vi "Kyriakakis_LabView_Software.vi"() -> ()   [LabVIEW 2012]
uses:
  <vilib>/MakerHub/LINX/LMH-LINX.lvlib
  <vilib>/MakerHub/LINX/Public/Peripherals/Digital/Digital Write N Chans.vi
panel:
  in  "Run Time           8":dbl min=0.0 step=60.0 format="%<%H:%M>t"
  in  "Run Time           7":dbl min=0.0 step=60.0 format="%<%H:%M>t"
  in  "Run Time           6":dbl min=0.0 step=60.0 format="%<%H:%M>t"
  in  "Run Time           5":dbl min=0.0 step=60.0 format="%<%H:%M>t"
  in  "Run Time           4":dbl min=0.0 step=60.0 format="%<%H:%M>t"
  in  "Run Time           3":dbl min=0.0 step=60.0 format="%<%H:%M>t"
  in  "Run Time           2":dbl min=0.0 step=60.0 format="%<%H:%M>t"
  in  "Run Time           1":dbl min=0.0 step=60.0 format="%<%H:%M>t"
  in  "Name/Notes":string
  in  "Pin #     8":u8=10 max=13 step=1
  out "Indicator         8":bool
  out "Cycle Time 8":dbl format="%<%H:%M>t"
  out "Frequency  8":dbl format="%#_3g mHz"
  in  "On/Off      8":bool
  out "On/Off indicator    8":bool
  in  "Time Off     8":dbl min=0.0 format="%#_4g min"
  in  "Time On    8":dbl min=0.0 format="%#_4g min"
  in  "Name/Notes":string
  in  "Pin #     7":u8=9 max=13 step=1
  out "Indicator         7":bool
  out "Cycle Time 7":dbl format="%<%H:%M>t"
  out "Frequency  7":dbl format="%#_3g mHz"
  in  "On/Off      7":bool
  out "On/Off indicator    7":bool
  in  "Time Off     7":dbl min=0.0 format="%#_2g min"
  in  "Time On    7":dbl min=0.0 format="%#_2g min"
  in  "Name/Notes":string
  in  "Pin #     6":u8=8 max=13 step=1
  out "Indicator         6":bool
  out "Cycle Time 6":dbl format="%<%H:%M>t"
  out "Frequency  6":dbl format="%#_3g mHz"
  in  "On/Off      6":bool
  out "On/Off indicator    6":bool
  in  "Time Off     6":dbl min=0.0 format="%#_2g min"
  in  "Time On    6":dbl min=0.0 format="%#_2g min"
  in  "Name/Notes":string
  in  "Pin #     5":u8=7 max=13 step=1
  out "Indicator         5":bool
  out "Cycle Time 5":dbl format="%<%H:%M>t"
  out "Frequency  5":dbl format="%#_3g mHz"
  in  "On/Off      5":bool
  out "On/Off indicator    5":bool
  in  "Time Off     5":dbl min=0.0 format="%#_2g min"
  in  "Time On    5":dbl min=0.0 format="%#_2g min"
  out "Connected":bool
  in  "?":bool
  in  "Name/Notes":string
  in  "Name/Notes":string
  in  "Name/Notes":string
  in  "Name/Notes":string
  in  "?":bool
  out "Run Complete":bool
  out "Time Has Elapsed":bool=TRUE
  out "Indicator         4":bool
  out "Cycle Time 4":dbl format="%<%H:%M>t"
  out "Frequency  4":dbl format="%#_3g mHz"
  in  "On/Off      4":bool
  out "On/Off indicator    4":bool
  in  "Time Off     4":dbl min=0.0 format="%#_2g min"
  in  "Time On    4":dbl min=0.0 format="%#_2g min"
  out "Indicator         3":bool
  out "Cycle Time 3":dbl format="%<%H:%M>t"
  out "Frequency  3":dbl format="%#_3g mHz"
  in  "On/Off      3":bool
  out "On/Off indicator    3":bool
  in  "Time Off     3":dbl min=0.0 format="%#_2g min"
  in  "Time On    3":dbl min=0.0 format="%#_2g min"
  in  "Pin #     4":u8=6 max=13 step=1
  in  "Pin #     3":i8=5 min=0 max=13 step=1
  in  "Pin #     2":u8=4 max=13 step=1
  out "Indicator         2":bool
  out "Cycle Time 2":dbl format="%<%H:%M>t"
  out "Frequency  2":dbl format="%#_3g mHz"
  in  "On/Off      2":bool
  out "On/Off indicator    2":bool
  in  "Time Off     2":dbl min=0.0 format="%#_2g min"
  in  "Time On    2":dbl min=0.0 format="%#_2g min"
  in  "Pin #     1":u8=3 max=13 step=1
  in  "Serial Port":refnum<visa-resource-name>
  out "Loop Rate (Hz)":u32
  out "Run Time":dbl format="%<%H:%M:%S>t"
  in  "Total Run Time \nH : M":dbl format="%<%M:%S>t"
  out "ACTIVE":bool
  in  "Start":bool
  out "Time till Start":dbl format="%<%H:%M:%S>t"
  in  "Start Delay\nH : M":dbl format="%<%M:%S>t"
  out "Total Elapsed Time":dbl format="%<%H:%M:%S>t"
  out "Indicator         1":bool
  out "Cycle Time 1":dbl format="%<%H:%M>t"
  out "Frequency  1":dbl format="%#_3g mHz"
  in  "On/Off      1":bool
  out "On/Off indicator    1":bool
  in  "Time Off     1":dbl min=0.0 format="%#_2g min"
  in  "Time On    1":dbl min=0.0 format="%#_2g min"
  # "Pin Controls:\nAll Time settings are given in Minutes\nKeep panel Off if not in use\nSelect pin you wish to use\nName/Notes can be edited for notes"
  # "Frequenices are in miliHertz (Cycles / 1000s)\nCycle Time is in Minutes\n% On is the Percentage of the On State\nIndicator indicaters if power is sent to light\nIf Individual Run times are 0, they default to total run time"
  # "Arduino Control Panel"
  # "Choose Serial Port from drop-down menu and click connect"
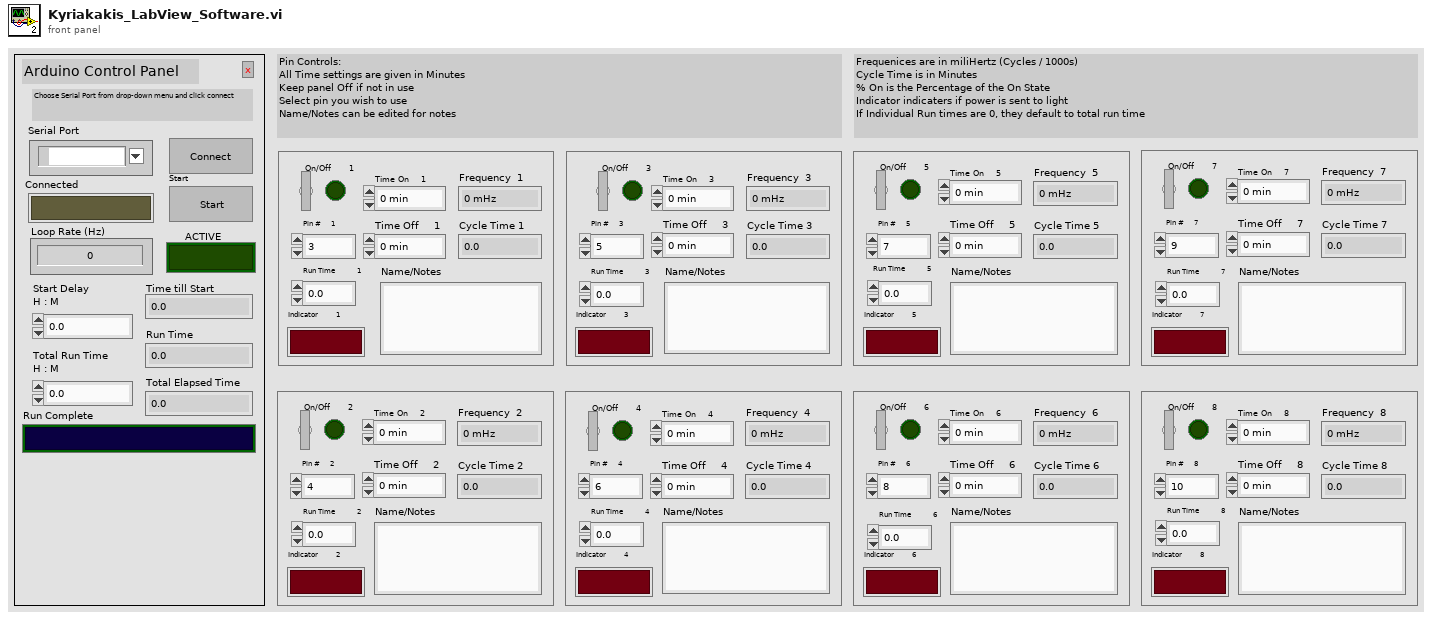
[diagram p1: front panel]
types:
  T1 = typedef "LMH-LINX.lvlib/LINX Ref.ctl" = cluster{"IO":T2, "Interface":T3, "LINX Device Config":T4}
  T2 = typedef "LMH-LINX.lvlib/Platform.ctl" = enum16{"Remote", "Local"}
  T3 = typedef "LMH-LINX.lvlib/Interface.ctl" = enum16{"Serial", "TCP"}
  T4 = typedef "LMH-LINX.lvlib/Device.lvlib/LINX Device Config.ctl" = cluster{"Interface":T3, "COM Port":refnum<visa-resource-name>, "TCP Configuration":T5, "Device Family":u8, "Device ID":u8, "Device Name":string, "TCP Ref":refnum<k5>, "Channels":T6}
  T5 = typedef "LMH-LINX.lvlib/Device.lvlib/TCP Config.ctl" = cluster{"IP Address":string, "Port":u16}
  T6 = typedef "LMH-LINX.lvlib/Channels.ctl" = cluster{"DI":u8[], "DO":u8[], "AI":u8[], "AO":u8[], "PWM":u8[], "QE":u8[], "UART":u8[], "I2C 2":u8[], "SPI":u8[], "CAN":u8[], "Servo":u8[], "AI Ref (V)":dbl, "AI Resolution (Bits)":u8, "AO Ref (V)":dbl, "AO Resolution (Bits)":u8}
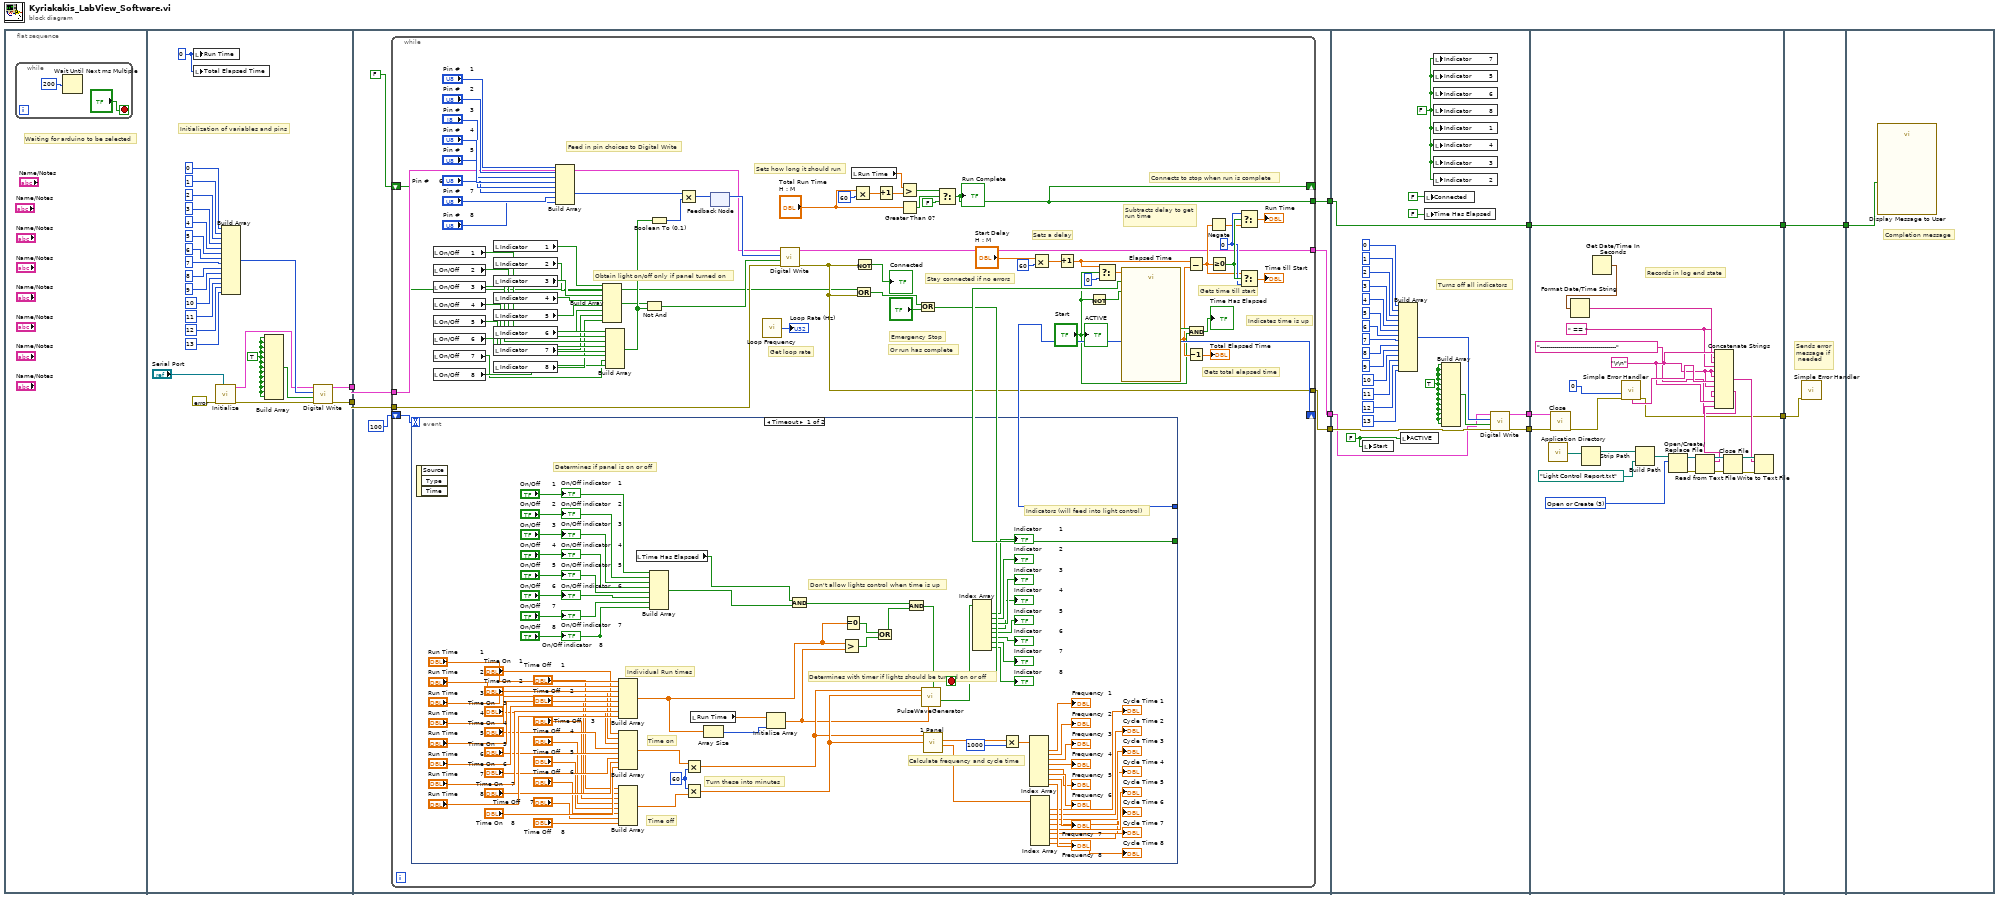
[diagram p0: block diagram]
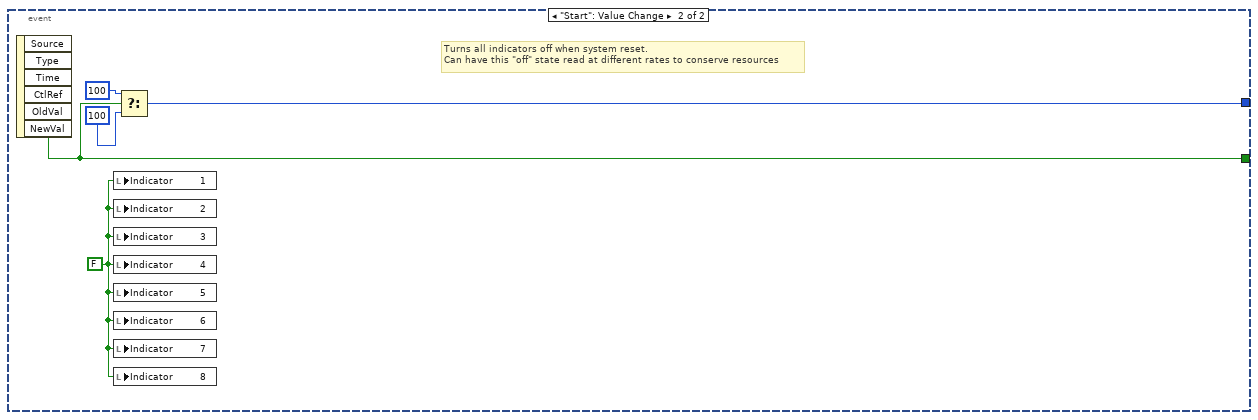
[diagram p2: hidden frame]
diagram:
  n1 = flat-sequence {
    tunnel: [w18] -> w7
    tunnel: [w17] -> w6
    tunnel: [w39] -> w11
    tunnel: [w40] -> w10
    tunnel: w7 -> [w44]
    tunnel: w6 -> [w43]
    tunnel: [w38] -> w5
    tunnel: w11 -> [w222]
    tunnel: w10 -> [w199]
    tunnel: [w220] -> w9
    tunnel: [w219] -> w8
    tunnel: w5 -> [w198]
    tunnel: [w198] -> w1
    tunnel: w9 -> [w248]
    tunnel: w8 -> [w247]
    tunnel: [w225] -> w4
    tunnel: [w224] -> w2
    tunnel: w1 -> [w224]
    tunnel: w4 -> [w250]
    tunnel: [w249] -> w3
    tunnel: w2 -> [w249]
    tunnel: w3 -> [w251]
    frame #0 {
      # "Waiting for arduino to be selected"
      n2 = while {
        stop <- "?" stop-if-true
        n3 = Wait Until Next ms Multiple(millisecond multiple=200) -> ()  [unwired: 1 out]
      }
    }
    frame #1 {
      w19 = TRUE
      w14 = 0
      # "Initialization of variables and pins"
      n4 = local write "Run Time"(w14) -> ()
      n5 = local write "Total Elapsed Time"(w14) -> ()
      n6 = call <vilib>:"Initialize.vi"("Serial Port"="Serial Port", "Error In"=errorcluster {"status"=FALSE, "code"=0, "source"=""}) -> ("Error Out"=w15:errorcluster, "LINX Resource"=w16:T1)  [unwired: 7 in, 1 out]
      n7 = Build Array(0, 1, 2, 3, 4, 5, 6, 7, 8, 9, 10, 11, 12, 13) -> (w20:i32[])
      n8 = Build Array(w19, w19, w19, w19, w19, w19, w19, w19, w19, w19, w19, w19, w19) -> (w35:bool[])
      n9 = call-poly <vilib>:"Digital Write.vi"("Error In"=w15, "Values"=w35, "DO Channels"=w20, "LINX Resource"=w16) -> ("Error Out"=w17:errorcluster, "LINX Resource"=w18:T1)  [unwired: 6 in]
    }
    frame #2 {
      n10 = while {
        shift-right: [w99] -> _
        shift-left: 100 -> [w98]
        tunnel: w43 -> [w87]
        tunnel: w44 -> [w49]
        tunnel: [w71] -> w39
        tunnel: [w86] -> w40
        shift-right: [w74] -> _
        shift-left: FALSE -> [w45]
        tunnel: [w74] -> w38
        stop <- w75 stop-if-true
        w108 = 0
        # "Or run has complete"
        # "Connects to stop when run is complete"
        # "Sets how long it should run"
        # "Gets time till start"
        # "Subtracts delay to get\nrun time"
        # "Sets a delay"
        # "Gets total elapsed time"
        # "Indicates time is up"
        # "Emergency Stop"
        # "Stay connected if no errors"
        # "Get loop rate"
        # "Obtain light on/off only if panel turned on"
        # "Feed in pin choices to Digital Write"
        n11 = event shown="[0] Timeout" {
          selector: _ -> [_ _]
          dyn-events: _ -> [_ _]
          timeout: w98 -> [_ _]
          tunnel: [_ w195] -> w99
          tunnel: [_ w194] -> w79
          event Timeout {
            w192 = 60
            # "Indicators (will feed into light control)"
            # "Determines with timer if lights should be turned on or off"
            # "Calculate frequency and cycle time"
            # "Turn these into minutes"
            # "Time off"
            # "Time on"
            # "Individual Run times"
            # "Don't allow lights control when time is up"
            # "Determines if panel is on or off"
            n12 = event-data() -> ()  [unwired: 1 in, 3 out]
            n13 = Build Array("Time On    1", "Time On    2", "Time On    3", "Time On    4", "Time On    5", "Time On    6", "Time On    7", "Time On    8") -> (w130:dbl[])
            n14 = Build Array("Run Time           1", "Run Time           2", "Run Time           3", "Run Time           4", "Run Time           5", "Run Time           6", "Run Time           7", "Run Time           8") -> (w118:dbl[])
            n15 = Build Array("Time Off     1", "Time Off     2", "Time Off     3", "Time Off     4", "Time Off     5", "Time Off     6", "Time Off     7", "Time Off     8") -> (w164:dbl[])
            n16 = local read "Time Has Elapsed"() -> (w121:bool)
            n17 = Build Array("On/Off      1", "On/Off      2", "On/Off      3", "On/Off      4", "On/Off      5", "On/Off      6", "On/Off      7", "On/Off      8") -> (w120:bool[])
            n18 = Multiply(x=w130, y=w192) -> (x*y=w145:dbl[])
            n19 = Multiply(x=w192, y=w164) -> (x*y=w146:dbl[])
            n20 = local read "Run Time"() -> (w142:dbl)
            n21 = Array Size(array=w118) -> (size(s)=w143:i32)
            n22 = Initialize Array(w142, w143) -> (w119:dbl[])
            n23 = And(x=w121, y=w120) -> (x .and. y?=w124:bool[])
            n24 = Greater?(x=w118, y=w119) -> (0:w190:bool[])
            n25 = Equal To 0?(x=w118) -> (x = 0?=w191:bool[])
            n26 = Or(x=w191, y=w190) -> (x .or. y?=w125:bool[])
            n27 = And(x=w124, y=w125) -> (x .and. y?=w144:bool[])
            n28 = call "PulseWaveGenerator.vi"("On/Off"=w144, "TIMER"=w119, "Time off (seconds)"=w146, "Time On (seconds)"=w145) -> ("Indicator"=w122:bool[])  [unwired: 6 in, 1 out]
            n29 = call "1 Panel.vi"("Time Off"=w146, "Time On"=w145) -> ("Cycle Time"=w155:dbl[], "Frequency"=w116:dbl[])  [unwired: 7 in, 1 out]
            n30 = Index Array(array=w122) -> (element #1=→"Indicator         1":bool, element #2=→"Indicator         2":bool, element #3=→"Indicator         3":bool, element #4=→"Indicator         4":bool, element #5=→"Indicator         5":bool, element #6=→"Indicator         6":bool, element #7=→"Indicator         7":bool, element #8=→"Indicator         8":bool)  [unwired: 8 in]
            n31 = Multiply(x=w116, y=1000) -> (x*y=w123:dbl[])
            n32 = Index Array(array=w123) -> (element #1=→"Frequency  1":dbl, element #2=→"Frequency  2":dbl, element #3=→"Frequency  3":dbl, element #4=→"Frequency  4":dbl, element #5=→"Frequency  5":dbl, element #6=→"Frequency  6":dbl, element #7=→"Frequency  7":dbl, element #8=→"Frequency  8":dbl)  [unwired: 8 in]
            n33 = Index Array(array=w155) -> (element #1=→"Cycle Time 1":dbl, element #2=→"Cycle Time 2":dbl, element #3=→"Cycle Time 3":dbl, element #4=→"Cycle Time 4":dbl, element #5=→"Cycle Time 5":dbl, element #6=→"Cycle Time 6":dbl, element #7=→"Cycle Time 7":dbl, element #8=→"Cycle Time 8":dbl)  [unwired: 8 in]
            "On/Off indicator    1" <- "On/Off      1"
            "On/Off indicator    2" <- "On/Off      2"
            "On/Off indicator    3" <- "On/Off      3"
            "On/Off indicator    4" <- "On/Off      4"
            "On/Off indicator    5" <- "On/Off      5"
            "On/Off indicator    6" <- "On/Off      6"
            "On/Off indicator    7" <- "On/Off      7"
            "On/Off indicator    8" <- "On/Off      8"
          }
          event "Start": Value Change {
            w193 = FALSE
            # "Turns all indicators off when system reset.\nCan have this \"off\" state read at different rates to conserve resources"
            n34 = event-data() -> ("NewVal"=w194:bool)  [unwired: 1 in, 5 out]
            n35 = local write "Indicator         1"(w193) -> ()
            n36 = local write "Indicator         2"(w193) -> ()
            n37 = local write "Indicator         3"(w193) -> ()
            n38 = local write "Indicator         4"(w193) -> ()
            n39 = local write "Indicator         5"(w193) -> ()
            n40 = local write "Indicator         6"(w193) -> ()
            n41 = local write "Indicator         7"(w193) -> ()
            n42 = local write "Indicator         8"(w193) -> ()
            n43 = Select(t=100, s=w194, f=100) -> (s? t:f=w195:i32)
          }
        }
        n44 = local read "On/Off      1"() -> (w70:bool)
        n45 = local read "On/Off      2"() -> (w67:bool)
        n46 = local read "On/Off      3"() -> (w68:bool)
        n47 = local read "On/Off      4"() -> (w69:bool)
        n48 = local read "On/Off      5"() -> (w61:bool)
        n49 = local read "On/Off      6"() -> (w60:bool)
        n50 = local read "On/Off      7"() -> (w52:bool)
        n51 = local read "On/Off      8"() -> (w53:bool)
        n52 = local read "Indicator         1"() -> (w97:bool)
        n53 = local read "Indicator         2"() -> (w94:bool)
        n54 = local read "Indicator         3"() -> (w96:bool)
        n55 = local read "Indicator         4"() -> (w95:bool)
        n56 = local read "Indicator         5"() -> (w59:bool)
        n57 = local read "Indicator         6"() -> (w58:bool)
        n58 = local read "Indicator         7"() -> (w55:bool)
        n59 = local read "Indicator         8"() -> (w54:bool)
        n60 = Build Array("Pin #     1", "Pin #     2", "Pin #     3", "Pin #     4", "Pin #     5", "Pin #     6", "Pin #     7", "Pin #     8") -> (w47:u8[])
        n61 = Build Array(w97, w94, w96, w95, w59, w58, w55, w54) -> (w48:bool[])
        n62 = Build Array(w70, w67, w68, w69, w61, w60, w52, w53) -> (w66:bool[])
        n63 = Not And(1:w66, 2:w48) -> (0:w51:bool[])
        n64 = Boolean To (0,1)(Boolean=w66) -> (0, 1=w46:i16[])
        n65 = Multiply(x=w47, y=w46) -> (x*y=w65:i16[])
        n66 = feedback-in #1(w65) -> ()
        n67 = feedback #1() -> (w64:i16[])  [unwired: 1 in]
        n68 = call <vilib>:"Loop Frequency.vi"() -> ("Loop Rate (Hz)"=→"Loop Rate (Hz)":u32)
        n69 = call-poly <vilib>:"Digital Write.vi"("Error In"=w87, "Values"=w51, "DO Channels"=w64, "LINX Resource"=w49) -> ("Error Out"=w71:errorcluster, "LINX Resource"=w86:T1)  [unwired: 6 in]
        n70 = local read "Run Time"() -> (w83:dbl)
        n71 = Multiply(x="Total Run Time \nH : M", y=60) -> (x*y=w93:dbl)
        n72 = Or(x=w45, y=w71) -> (x .or. y?=w89:bool)
        n73 = Not(x=w71) -> (.not. x?=→"Connected":bool)
        n74 = Increment(x=w93) -> (x+1=w92:dbl)
        n75 = Greater?(x=w83, y=w92) -> (0:w105:bool)
        n76 = Greater Than 0?(x="Total Run Time \nH : M") -> (x > 0?=w76:bool)
        n77 = Or(x=w89, y="?") -> (x .or. y?=w75:bool)
        n78 = Select(t=w105, s=w76, f=FALSE) -> (s? t:f=w74:bool)
        "Run Complete" <- w74
        n79 = Multiply(x="Start Delay\nH : M", y=60) -> (x*y=w90:dbl)
        n80 = Increment(x=w90) -> (x+1=w82:dbl)
        n81 = Not(x="Start") -> (.not. x?=w78:bool)
        n82 = Select(t=w82, s="Start", f=0) -> (s? t:f=w81:dbl)
        n83 = call "Elapsed Time"("Time Target (s)"=w81, "Reset"=w79, "Auto Reset"=w78) -> ("Elapsed Time (s)"=w84:dbl, "Time has Elapsed"=w100:bool)  [unwired: 9 in, 6 out]
        n84 = Subtract(x=w82, y=w84) -> (x-y=w106:dbl)
        n85 = Decrement(x=w84) -> (x-1=→"Total Elapsed Time":dbl)
        n86 = And(x=w100, y="Start") -> (x .and. y?=→"Time Has Elapsed":bool)
        n87 = Negate(x=w106) -> (-x=w107:dbl)
        n88 = Greater Or Equal To 0?(x=w106) -> (x >= 0?=w110:bool)
        n89 = Select(t=w108, s=w110, f=w107) -> (s? t:f=→"Run Time":dbl)
        n90 = Select(t=w106, s=w110, f=w108) -> (s? t:f=→"Time till Start":dbl)
        "ACTIVE" <- "Start"
      }
    }
    frame #3 {
      w218 = FALSE
      w201 = TRUE
      w200 = FALSE
      # "Turns off all indicators"
      n91 = local write "Start"(w218) -> ()
      n92 = Build Array(0, 1, 2, 3, 4, 5, 6, 7, 8, 9, 10, 11, 12, 13) -> (w202:i32[])
      n93 = local write "ACTIVE"(w218) -> ()
      n94 = local write "Connected"(FALSE) -> ()
      n95 = local write "Time Has Elapsed"(FALSE) -> ()
      n96 = local write "Indicator         7"(w200) -> ()
      n97 = local write "Indicator         5"(w200) -> ()
      n98 = local write "Indicator         6"(w200) -> ()
      n99 = local write "Indicator         8"(w200) -> ()
      n100 = local write "Indicator         1"(w200) -> ()
      n101 = local write "Indicator         4"(w200) -> ()
      n102 = local write "Indicator         3"(w200) -> ()
      n103 = local write "Indicator         2"(w200) -> ()
      n104 = Build Array(w201, w201, w201, w201, w201, w201, w201, w201, w201, w201, w201, w201, w201) -> (w221:bool[])
      n105 = call-poly <vilib>:"Digital Write.vi"("Error In"=w222, "Values"=w221, "DO Channels"=w202, "LINX Resource"=w199) -> ("Error Out"=w219:errorcluster, "LINX Resource"=w220:T1)  [unwired: 6 in]
    }
    frame #4 {
      w228 = " == "
      w238 = u16 3 items=["Open", "Replace", "Create", "Open or Create", "Create or Replace", "Create or Replace with Confirm", ""]
      w227 = "--------------------------------------"
      w230 = "\r\n"
      # "Records in log end state"
      n106 = call <vilib>:"Application Directory.vi"() -> ("Application Directory"=w243:path)
      n107 = call <vilib>:"Close.vi"("Error In"=w247, "LINX Resource"=w248) -> ("Error Out"=w246:errorcluster)  [unwired: 9 in]
      n108 = Strip Path(path=w243) -> (stripped path=w245:path)  [unwired: 1 out]
      n109 = Get Date/Time In Seconds() -> (seconds since 1Jan1904=w242:timestamp)
      n110 = Format Date/Time String(seconds (now)=w242) -> (date/time string=w229:string)  [unwired: 2 in]
      n111 = call <vilib>:"Simple Error Handler.vi"("type of dialog (OK msg:1)"=0, "error in (no error)"=w246) -> ("error out"=w225:errorcluster, "message"=w233:string)  [unwired: 3 in, 3 out]
      n112 = Build Path(base path=w245, name or relative path=path "Light Control Report.txt") -> (appended path=w241:path)
      n113 = Open/Create/Replace File(file path (use dialog)=w241, operation (0:open)=w238) -> (refnum out=w239:refnum<file>, error out=w240:errorcluster)  [unwired: 4 in, 1 out]
      n114 = Read from Text File(file (use dialog)=w239, error in=w240) -> (refnum out=w237:refnum<file>, text=w232:string, error out=w236:errorcluster)  [unwired: 2 in, 1 out]
      n115 = Concatenate Strings(w230, w228, w229, w228, w230, w230, w233, w230, w227, w227, w230, w232) -> (w231:string)
      n116 = Close File(refnum=w237, error in=w236) -> (path=w235:path, error out=w234:errorcluster)
      n117 = Write to Text File(file (use dialog)=w235, text=w231, error in=w234) -> ()  [unwired: 1 in, 3 out]
    }
    frame #5 {
      # "Sends error\nmessage if\n needed"
      n118 = call <vilib>:"Simple Error Handler.vi"("error in (no error)"=w250) -> ()  [unwired: 4 in, 5 out]
    }
    frame #6 {
      # "Completion message"
      n119 = call "Display Message to User"("Enable"=w251) -> ()  [unwired: 9 in, 2 out]
    }
  }
